vi "RequestDestroy.vi"(8 "ErrorIn":errorcluster, 11 "ReferenceIn":refnum<class "TemplateGUI.lvclass">) -> (0 "ErrorOut":errorcluster, 3 "ReferenceOut":refnum<class "TemplateGUI.lvclass">)   [LabVIEW 2021, in "TemplateGUIOpenGDSActiveObject.lvlib" / "TemplateGUI.lvclass"]
uses:
  TemplateGUI.lvclass
  3fbc1877-3ae8-4aff-a423-cebf9be5a0b1.vi
  MainGUIRepository.vi
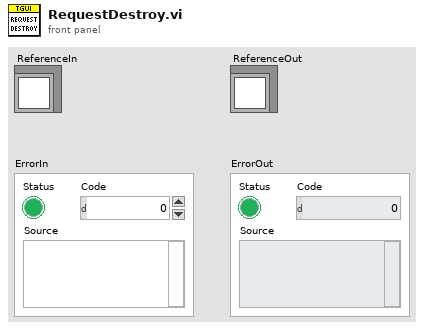
[diagram p1: front panel]
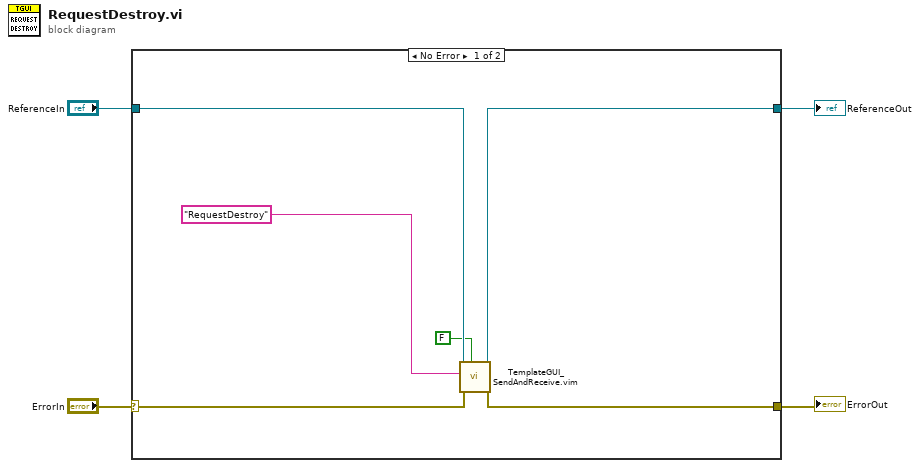
[diagram p0: block diagram]
diagram:
  n1 = case shown="No Error" "ErrorIn" {
    selector: "ErrorIn" -> [w10 w12]
    tunnel: [w9 w12] -> w3
    tunnel: [w7 w11] -> w1
    tunnel: "ReferenceIn" -> [w8 w11]
    frame No Error {
      n2 = call "TemplateGUI_SendAndReceive.vim"("ShouldWeWaitForResponse"=FALSE, "ErrorIn"=w10, "Command"="RequestDestroy", "ReferenceIn"=w8) -> ("ErrorOut"=w9:errorcluster, "ReferenceOut"=w7:refnum<class "TemplateGUI.lvclass">)  [unwired: 5 in, 1 out]
    }
    frame Error {
    }
  }
  "ErrorOut" <- w3
  "ReferenceOut" <- w1
